vi "BK Precision 8500B Series Monitor Input.vi"() -> ()   [LabVIEW 2019]
doc: "Exemplifies monitoring the input voltage and current in constant current mode."
uses:
  <instrlib>/BK Precision 8500B Series/BK Precision 8500B Series.lvlib
panel:
  in  "CC Current (0)":dbl min=0.0 max=240.0 step=1.0 format="%#.3f"
  out "Current":dbl format="%_6g"
  out "Voltage":dbl format="%_6f"
  in  "?":bool
  in  "VISA resource name":refnum<visa-resource-name>
  in  "Serial Configuration":cluster{"Baud Rate":u32}={"Baud Rate"=9600} {"Baud Rate" items=["300"=300, "600"=600, "1200"=1200, "2400"=2400, "4800"=4800, "9600"=9600, "19200"=19200]}
  # "(c) 2019 B&K Precision Corporation.  ALL RIGHTS RESERVED."
  # "A"
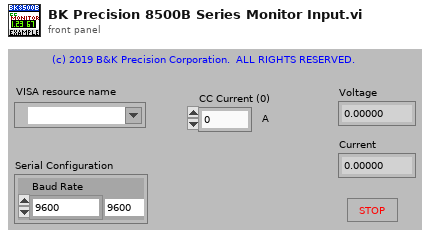
[diagram p1: front panel]
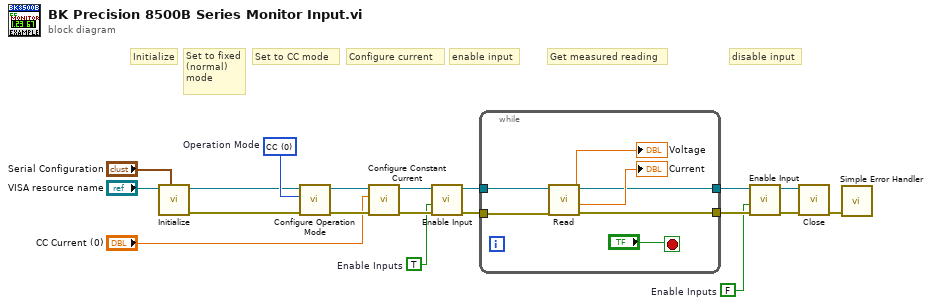
[diagram p0: block diagram]
diagram:
  w3 = u16 0 items=["CC", "CV", "CR", "CW", "CZ"]  # Operation Mode
  w5 = TRUE  # Enable Inputs
  w6 = FALSE  # Enable Inputs
  # "disable input"
  # "Get measured reading"
  # "enable input"
  # "Configure current"
  # "Set to CC mode"
  # "Set to fixed\n(normal)\nmode"
  # "Initialize"
  n1 = call <instrlib>:"Initialize.vi"("Serial Configuration"="Serial Configuration", "VISA resource name"="VISA resource name") -> ("error out"=w1:errorcluster, "VISA resource name out"=w2:refnum<visa-resource-name>)  [unwired: 8 in]
  n2 = call <instrlib>:"Configure Operation Mode.vi"("error in (no error)"=w1, "Operation Mode (0:CC)"=w3, "VISA resource name"=w2) -> ("error out"=w13:errorcluster, "VISA resource name out"=w14:refnum<visa-resource-name>)  [unwired: 7 in]
  n3 = call <instrlib>:"Configure Constant Current.vi"("error in (no error)"=w13, "CC Current (0)"="CC Current (0)", "VISA resource name"=w14) -> ("error out"=w11:errorcluster, "VISA resource name out"=w12:refnum<visa-resource-name>)  [unwired: 7 in]
  n4 = call <instrlib>:"Enable Input.vi"("error in (no error)"=w11, "Enable Input (F: False)"=w5, "VISA resource name"=w12) -> ("error out"=w9:errorcluster, "VISA resource name out"=w10:refnum<visa-resource-name>)  [unwired: 7 in]
  n5 = while {
    tunnel: w10 -> [w24]
    tunnel: w9 -> [w23]
    tunnel: [w22] -> w7
    tunnel: [w21] -> w8
    stop <- "?" stop-if-true
    n6 = call <instrlib>:"Read.vi"("error in (no error)"=w23, "VISA resource name"=w24) -> ("error out"=w22:errorcluster, "Current"=→"Current":dbl, "Voltage"=→"Voltage":dbl, "VISA resource name out"=w21:refnum<visa-resource-name>)  [unwired: 6 in]
  }
  n7 = call <instrlib>:"Enable Input.vi"("error in (no error)"=w7, "Enable Input (F: False)"=w6, "VISA resource name"=w8) -> ("error out"=w16:errorcluster, "VISA resource name out"=w15:refnum<visa-resource-name>)  [unwired: 7 in]
  n8 = call <instrlib>:"Close.vi"("error in (no error)"=w16, "VISA resource name"=w15) -> ("error out"=w17:errorcluster)  [unwired: 9 in]
  n9 = call <vilib>:"Simple Error Handler.vi"("error in (no error)"=w17) -> ()  [unwired: 4 in, 5 out]
